vi "FGV.vi"(8 "error in (no error)":errorcluster, 10 "Mode (Update)":enum16{"Update", "Init"}(ring)) -> (0 "error out":errorcluster, 2 "Iterations":u32)   [LabVIEW 2013]
doc: "Use this template to build a VI to use as a subVI."
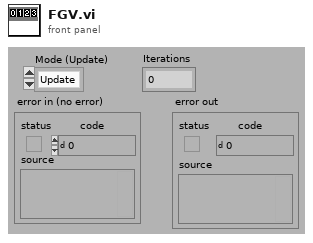
[diagram p1: front panel]
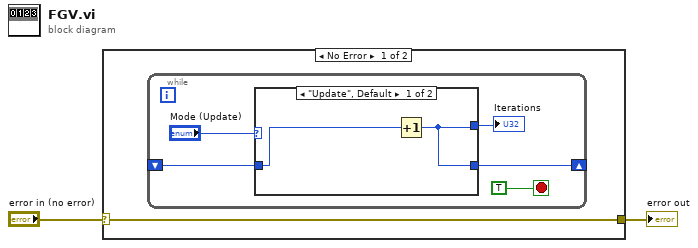
[diagram p0: block diagram]
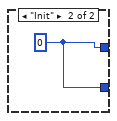
[diagram p2: hidden frame]
diagram:
  n1 = case shown="No Error" "error in (no error)" {
    selector: "error in (no error)" -> [w3 w12]
    tunnel: [w3 w12] -> w1
    frame No Error {
      n2 = while {
        shift-right: [w4] -> _
        shift-left: _ -> [w7]
        stop <- TRUE stop-if-true
        n3 = case shown="\"Update\", Default" "Mode (Update)" {
          tunnel: w7 -> [w10 _]
          tunnel: [w9 w11] -> w6
          tunnel: [w9 w11] -> w4
          frame "Update", Default {
            n4 = Increment(x=w10) -> (x+1=w9:u32)
          }
          frame "Init" {
            w11 = u32 0
          }
        }
        "Iterations" <- w6
      }
    }
    frame Error {
    }
  }
  "error out" <- w1
